vi "Flip 2D Array.vi"(11 "Hours":string[][](array[string])) -> (3 "Hours Flipped":string[][](array[string]))   [LabVIEW 2015]
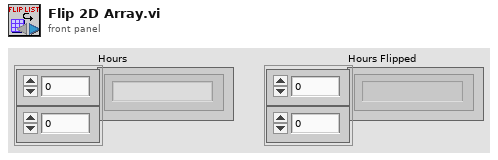
[diagram p1: front panel]
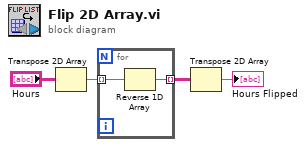
[diagram p0: block diagram]
diagram:
  n1 = Transpose 2D Array(2D array="Hours") -> (transposed array=w2:string[][])
  n2 = for {
    tunnel: w2 -> [w6] mode=indexing
    tunnel: [w5] -> w1 mode=indexing
    n3 = Reverse 1D Array(array=w6) -> (reversed array=w5:string[])
  }
  n4 = Transpose 2D Array(2D array=w1) -> (transposed array=→"Hours Flipped":string[][])
